vi "HELP Command.vi"(8 "error in (no error)":errorcluster, 10 "Command":string, 11 "Instrument in":refnum<class "Instrument.lvclass">) -> (0 "error out":errorcluster, 2 "HELP out":string, 3 "Instrument in":refnum<class "Instrument.lvclass">)   [LabVIEW 2019, in "Instrument.lvlib" / "Instrument.lvclass"]
doc: "Send \"HELP\" command to get API supported by remote Instrument."
uses:
  Instrument.lvclass
  Typedefs/Instrument.Commands--Enum.ctl
  HELP--Cluster.ctl
  13847043-707b-4050-995d-7bfd780093fb.vi
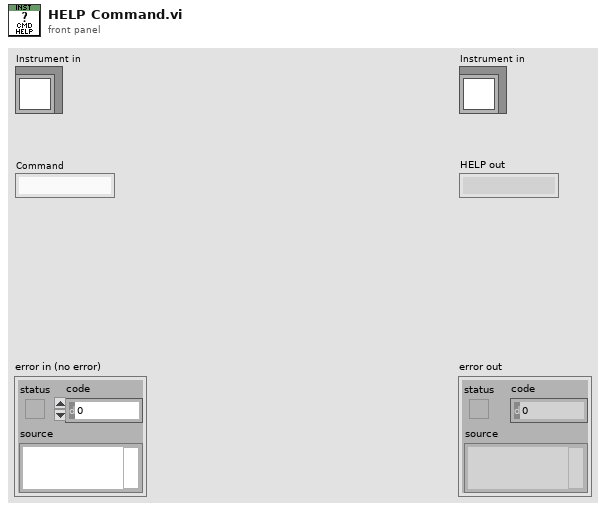
[diagram p1: front panel]
types:
  T1 = typedef "Instrument.lvlib/Instrument.lvclass/HELP--Cluster.ctl" = cluster{"Command":string}
  T2 = typedef "Instrument.lvlib/Instrument.lvclass/Instrument.Commands--Enum.ctl" = enum16{"ACK", "HELP", "IDN", "getAll", "getAllData"}
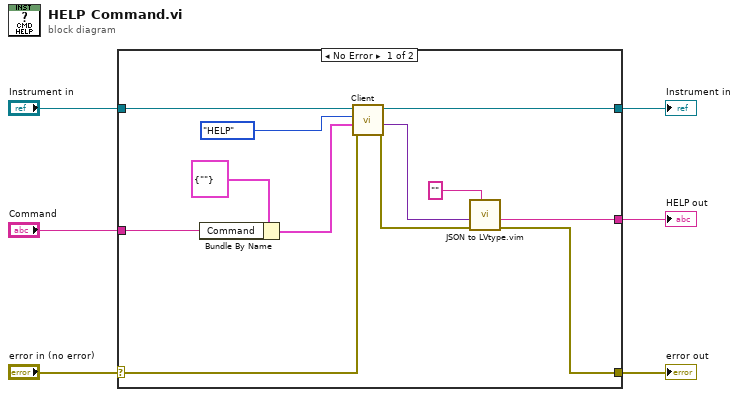
[diagram p0: block diagram]
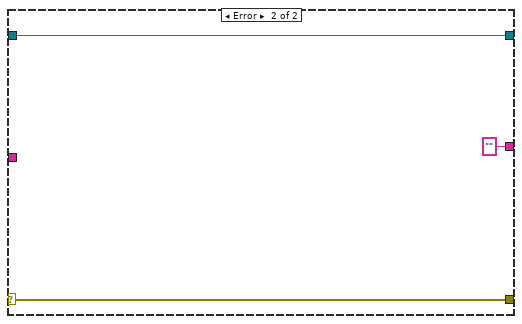
[diagram p2: hidden frame]
diagram:
  n1 = case shown="No Error" "error in (no error)" {
    selector: "error in (no error)" -> [w16 w21]
    tunnel: [w9 w21] -> w5
    tunnel: [w18 w20] -> w3
    tunnel: "Instrument in" -> [w17 w20]
    tunnel: "Command" -> [w13 _]
    tunnel: [w7 "" ("Data out")] -> w1
    frame No Error {
      n2 = Bundle By Name(cluster=T1 {"Command"=""}, "Command"=w13) -> (w12:T1)
      n3 = call-dynamic "Client.vi"("error in (no error)"=w16, "Data in"=w12, "Command in"=Instrument.Commands--Enum."HELP" ("Commands"), "Instrument in"=w17) -> ("error out"=w10:errorcluster, "Data out"=w11:variant, "Instrument out"=w18:refnum<class "Instrument.lvclass">)  [unwired: 4 in, 1 out]
      n4 = call "JSON to LVtype.vim"("type"="", "error in (no error)"=w10, "JSON Data in"=w11) -> ("error out"=w9:errorcluster, "Data out"=w7:string)  [unwired: 7 in]
    }
    frame Error {
    }
  }
  "error out" <- w5
  "Instrument in" <- w3
  "HELP out" <- w1
